vi "Detailed Complimentary (Mark Stangl's conflicted copy 2012-10-25).vi"() -> ()   [LabVIEW 2012]
panel:
  out "Temp C":dbl=1001.8
  out "Press mB":dbl=1001.8
  in  "?":bool
  in  "System Status":cluster{bool, bool, bool, bool, bool, bool}={TRUE, TRUE, TRUE, TRUE, TRUE, TRUE}
  out "Time Stamp":timestamp
  out "Altitude 3":dbl=88890.0
  in  "Confirm Now":bool
  in  "Notes":string
  in  "Datlog File":path
  out "Waveform Graph 2":dbl[](graph)
  out "Waveform Graph":dbl[](graph)
  in  "RUN":bool=TRUE
  in  "Altitude 2":dbl=88890.0
  out "Altitude":dbl=88888.0
  in  "Cluster":T1
  # "M\ne\nt\ne\nr\ns"
  # "WARNING"
  # "%"
  # "CO2"
  # "HOLD"
  # "OFF"
  # "Set-up"
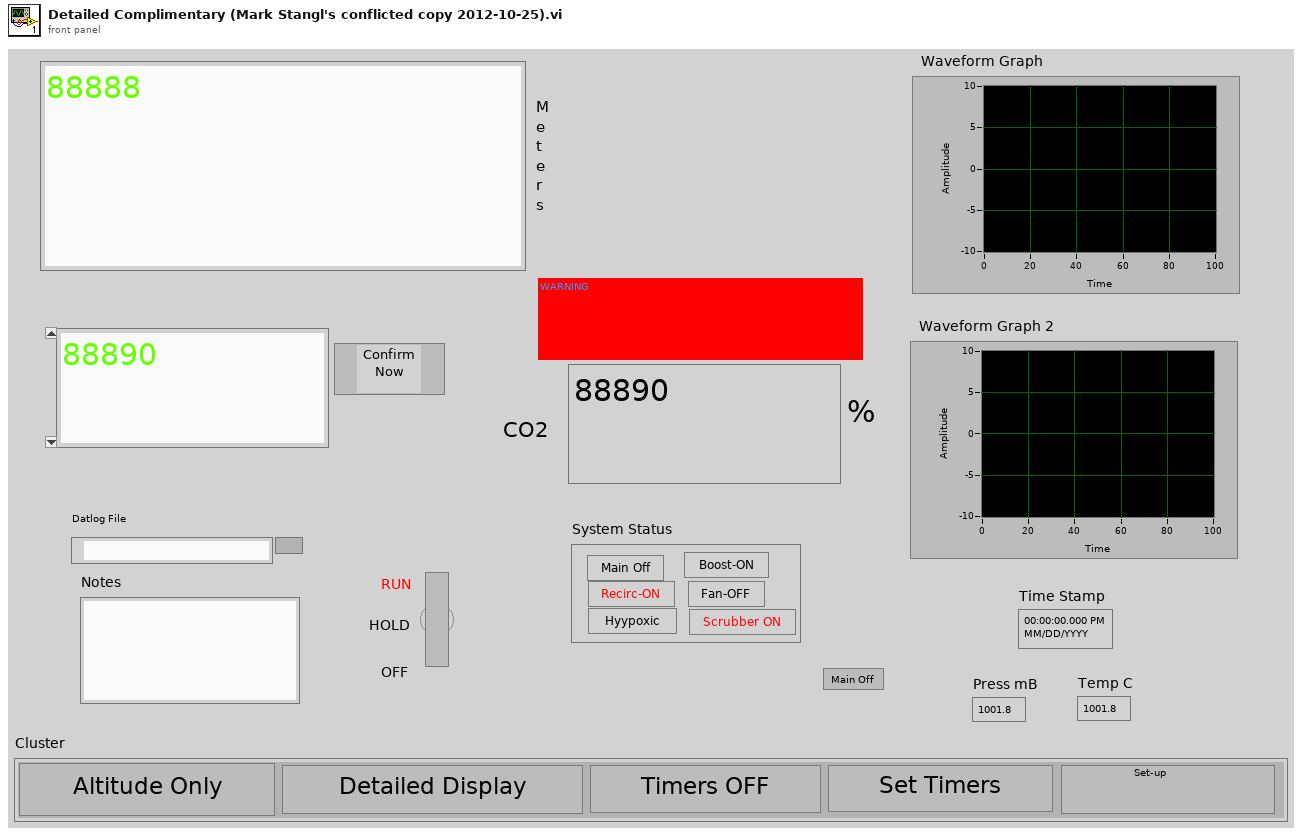
[diagram p1: front panel]
types:
  T1 = cluster{"OK Button":bool, "OK Button 2":bool, "OK Button":bool, "OK Button 4":bool, "OK Button 3":bool}
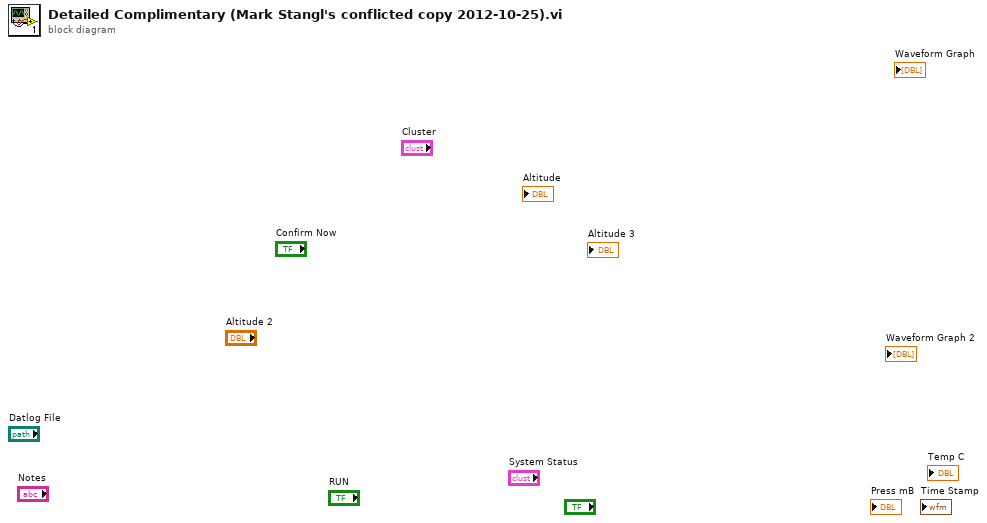
[diagram p0: block diagram]
diagram:
